vi "muti channel change.vi"(9 "Array - Numeric":dbl[](array[numeric]), 10 "?":T1(array[cluster]) {"Terminal Configuration" items=["default"=-1, "RSE"=10083, "NRSE"=10078, "Differential"=10106, "Pseudodifferential"=12529]}, 11 "data in":waveform(dbl)[](array[waveform])) -> (3 "data out":waveform(dbl)[](array[waveform]))   [LabVIEW 2024]
panel:
  out "empty channel":i32
  in  "element":waveform(dbl)
  out "current channel":i32
  out "current begin channel":i32
  out "data size":i32
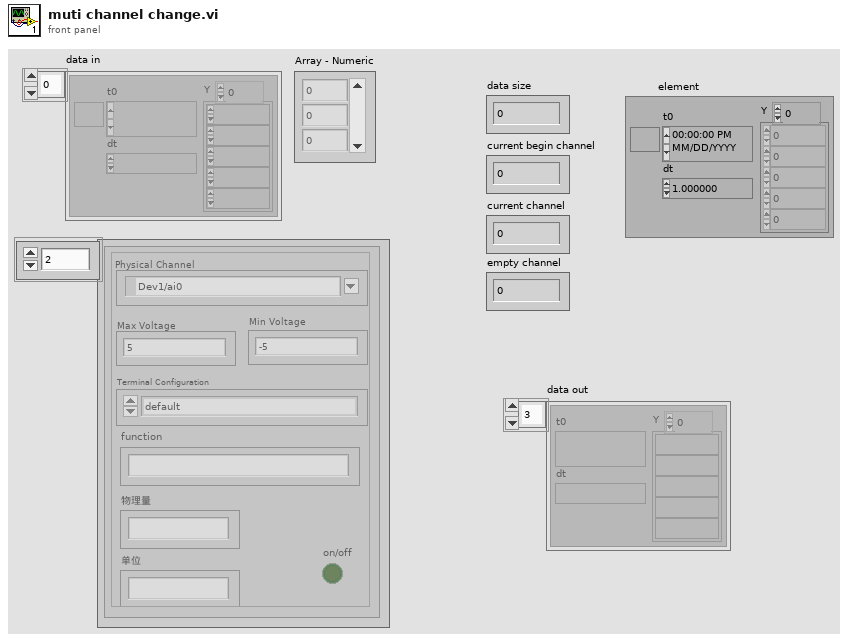
[diagram p1: front panel]
types:
  T1 = cluster{"Terminal Configuration":i32, "Min Voltage":dbl, "Physical Channel":tag, "Max Voltage":dbl, "function":string, "on/off":bool, "物理量":string, "单位":string}[]
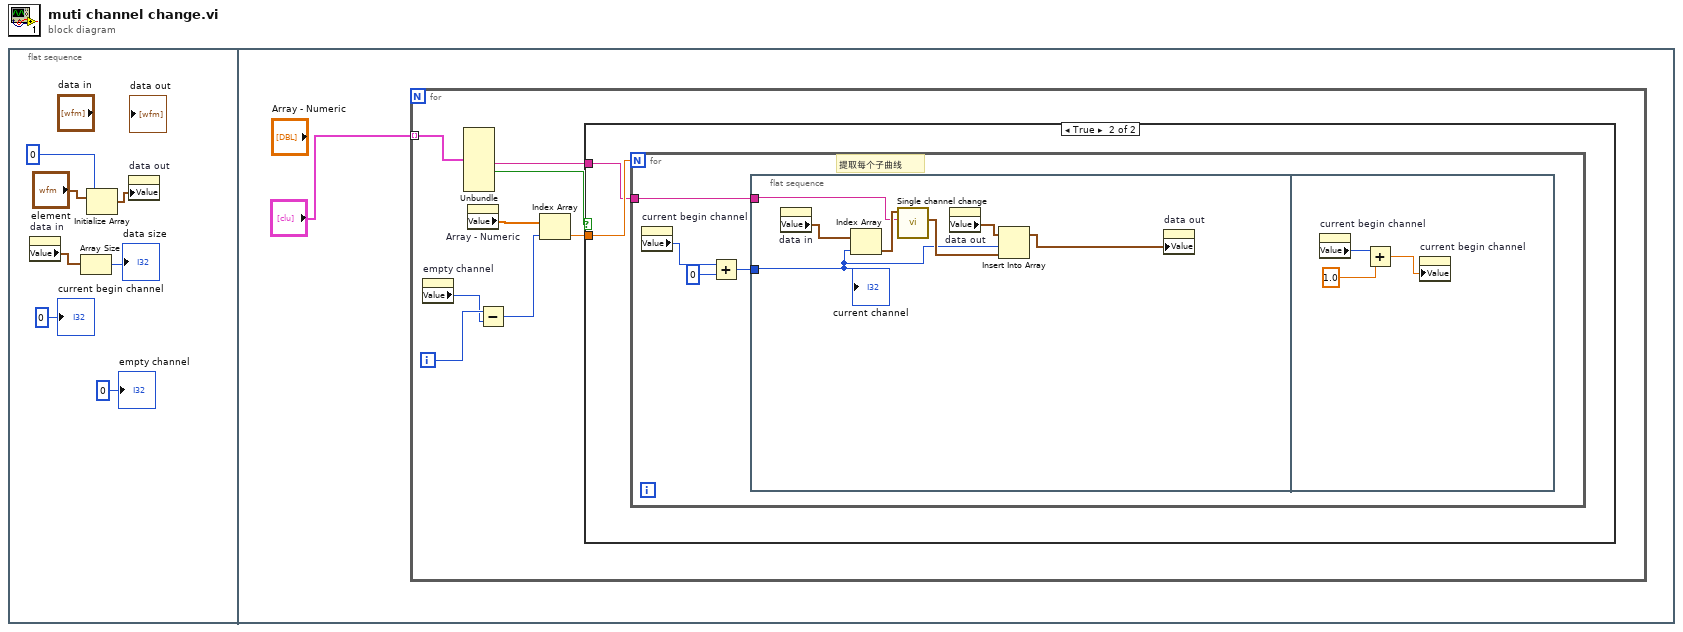
[diagram p0: block diagram]
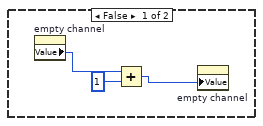
[diagram p2: hidden frame]
diagram:
  n1 = flat-sequence {
    frame #0 {
      n2 = property on="data in" class="Arr (strict)"() -> ("Value"=w7:waveform(dbl)[])  [unwired: 2 in, 2 out]
      n3 = Array Size(array=w7) -> (size(s)=→"data size":i32)
      n4 = Initialize Array("element", 0 ("dimension size")) -> (w2:waveform(dbl)[])
      n5 = property on="data out" class="Arr (strict)"("Value"=w2) -> ()  [unwired: 2 in, 2 out]
      "current begin channel" <- 0 ("current child channel")
      "empty channel" <- 0 ("empty channel")
    }
    frame #1 {
      n6 = for {
        tunnel: "?" -> [w14] mode=indexing
        i -> [w11]
        n7 = property on="empty channel" class="DigNum (strict)"() -> ("Value"=w10:i32)  [unwired: 2 in, 2 out]
        n8 = Unbundle(w14) -> ("function"=w13:string, "on/off"=w12:bool)  [unwired: 6 out]
        n9 = property on="Array - Numeric" class="Arr (strict)"() -> ("Value"=w16:dbl[])  [unwired: 2 in, 2 out]
        n10 = Subtract(x=w11, y=w10) -> (x-y=w9:i32)
        n11 = Index Array(array=w16, index=w9) -> (element=w15:dbl)
        n12 = case shown="True" w12 {
          tunnel: w15 -> [_ w21]
          tunnel: w13 -> [_ w20]
          frame False {
            n13 = property on="empty channel" class="DigNum (strict)"() -> ("Value"=w19:i32)  [unwired: 2 in, 2 out]
            n14 = Add(x=w19, y=1) -> (x+y=w17:i32)
            n15 = property on="empty channel" class="DigNum (strict)"("Value"=w17) -> ()  [unwired: 2 in, 2 out]
          }
          frame True {
            n16 = for {
              N: w21 -> [_]
              tunnel: w20 -> [w23]
              # "提取每个子曲线"
              n17 = property on="current begin channel" class="DigNum (strict)"() -> ("Value"=w25:i32)  [unwired: 2 in, 2 out]
              n18 = Add(x=w25, y=0) -> (x+y=w24:i32)
              n19 = flat-sequence {
                tunnel: w24 -> [w27]
                tunnel: w23 -> [w30]
                frame #0 {
                  n20 = property on="data in" class="Arr (strict)"() -> ("Value"=w32:waveform(dbl)[])  [unwired: 2 in, 2 out]
                  n21 = Index Array(array=w32, index=w27) -> (element=w31:waveform(dbl))
                  n22 = call "Single channel change.vi"("String"=w30, "element in"=w31) -> ("element out"=w28:waveform(dbl))  [unwired: 9 in]
                  n23 = property on="data out" class="Arr (strict)"() -> ("Value"=w29:waveform(dbl)[])  [unwired: 2 in, 2 out]
                  n24 = Insert Into Array(array=w29, index=w27, new element=w28) -> (w26:waveform(dbl)[])
                  n25 = property on="data out" class="Arr (strict)"("Value"=w26) -> ()  [unwired: 2 in, 2 out]
                  "current channel" <- w27
                }
                frame #1 {
                  n26 = property on="current begin channel" class="DigNum (strict)"() -> ("Value"=w34:i32)  [unwired: 2 in, 2 out]
                  n27 = Add(x=w34, y=1.0) -> (x+y=w33:dbl)
                  n28 = property on="current begin channel" class="DigNum (strict)"("Value"=w33) -> ()  [unwired: 2 in, 2 out]
                }
              }
            }
          }
        }
      }
    }
  }
